vi "Read Configuration Data.vi"(8 "Error In":errorcluster) -> (0 "Error Out":errorcluster, 3 "MHL Configuration":T1)   [LabVIEW 2015]
uses:
  controls/MHL Configuration.ctl
  Boiler System Globals.vi
  <vilib>/Utility/config.llb/NI_LVConfig.lvlib
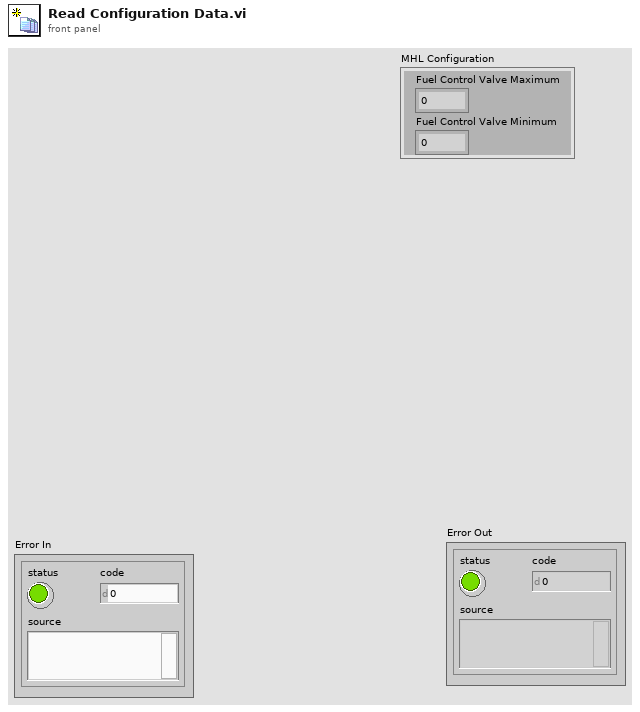
[diagram p1: front panel]
types:
  T1 = typedef "MHL Configuration.ctl" = cluster{"Fuel Control Valve Maximum":dbl, "Fuel Control Valve Minimum":dbl}
  T2 = typedef "NI_LVConfig.lvlib/Config Data RefNum.ctl" = refnum<k1>
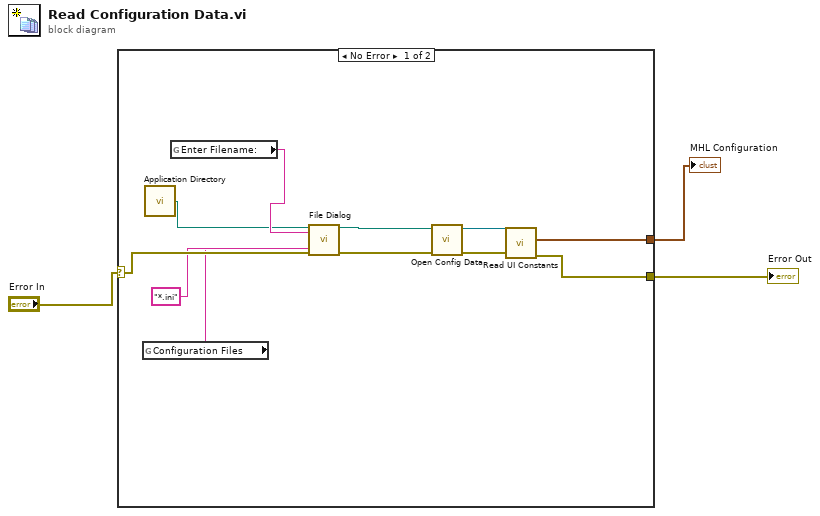
[diagram p0: block diagram]
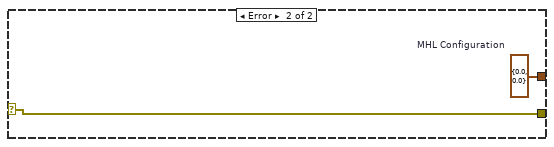
[diagram p2: hidden frame]
diagram:
  n1 = case shown="No Error" "Error In" {
    selector: "Error In" -> [w14 w16]
    tunnel: [w5 w16] -> w2
    tunnel: [w4 w15] -> w1
    frame No Error {
      n2 = global read "Boiler System Globals.vi" "Configuration Files"() -> (w11:string)
      n3 = call <vilib>:"Application Directory.vi"() -> ("Application Directory"=w10:path)
      n4 = global read "Boiler System Globals.vi" "Enter Filename:"() -> (w13:string)
      n5 = call "File Dialog"("start path"=w10, "prompt"=w13, "error in"=w14, "pattern (all files)"="*.ini" ("pattern label"), "pattern label"=w11) -> ("selected path"=w8:path, "error out"=w9:errorcluster)  [unwired: 7 in, 2 out]
      n6 = call <vilib>:"Open Config Data.vi"("error in (no error)"=w9, "configuration file path"=w8) -> ("error out"=w7:errorcluster, "refnum"=w6:T2)  [unwired: 7 in, 1 out]
      n7 = call "Read UI Constants.vi"("Error In"=w7, "refnum"=w6) -> ("Error Out"=w5:errorcluster, "output cluster"=w4:T1)  [unwired: 7 in, 1 out]
    }
    frame Error {
      w15 = T1 {"Fuel Control Valve Maximum"=0.0, "Fuel Control Valve Minimum"=0.0}  # MHL Configuration
    }
  }
  "Error Out" <- w2
  "MHL Configuration" <- w1
